vi "Lookup Channels.vi"(8 "error in (no error)":errorcluster, 11 "HTTP Command Bridge in":refnum<class "HTTP Command Bridge.lvclass">) -> (0 "error out":errorcluster, 3 "HTTP Command Bridge out":refnum<class "HTTP Command Bridge.lvclass">)   [LabVIEW 2020, in "Volatus.lvlib" / "HTTP Command Bridge.lvclass"]
uses:
  HTTP Command Bridge.lvclass
  HTTP Command Bridge.lvclass/HTTP Command Bridge.ctl
  Module/Module.lvclass
  VolatusAPI/VolatusAPI.lvclass
  Command Dest.ctl
  MessageQ/MessageQ.lvclass
  Command Info.ctl
  C:/dev/lv20CE/relink/lv-volatus/Volatus/Module/Module.lvclass
  C:/dev/lv20CE/relink/lv-volatus/Volatus/HTTP Command Bridge/HTTP Command Bridge.lvclass
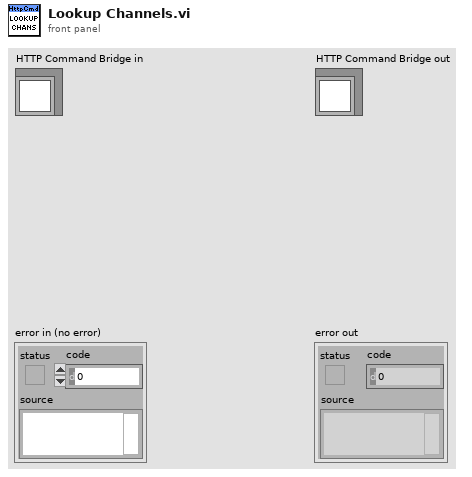
[diagram p1: front panel]
types:
  T1 = typedef "Volatus.lvlib/HTTP Command Bridge.lvclass/Command Info.ctl" = cluster{"Destination":T2, "Local Q":refnum<class "MessageQ.lvclass">, "Target":string, "Task":string}
  T2 = typedef "Volatus.lvlib/HTTP Command Bridge.lvclass/Command Dest.ctl" = enum16{"Local", "Remote"}
  T3 = typedef "VectoConfig.lvlib/Channel Info.ctl" = cluster{"Name":string, "Group":string, "Owning Node":string, "Owning Task":string, "Resource":string}
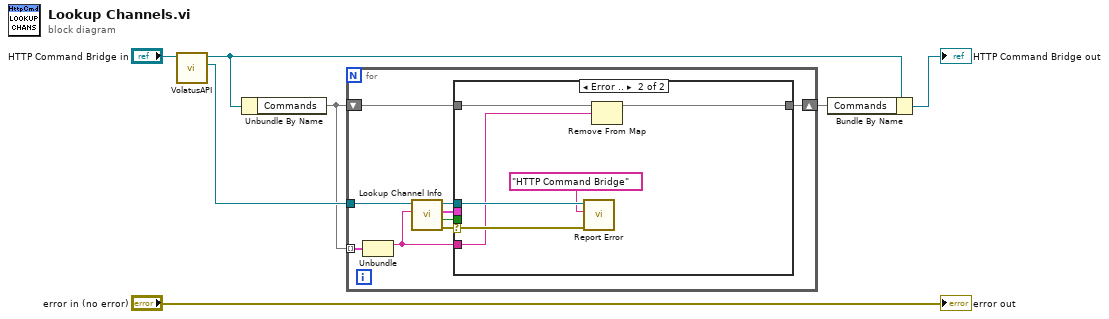
[diagram p0: block diagram]
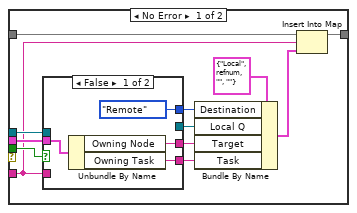
[diagram p2: hidden frame]
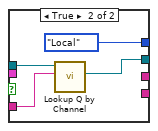
[diagram p3: hidden frame]
diagram:
  n1 = call "VolatusAPI.vi"("Module in"="HTTP Command Bridge in") -> ("VolatusAPI"=w6:refnum<class "VolatusAPI.lvclass">, "Module out"=w4:refnum<class "HTTP Command Bridge.lvclass">)  [unwired: 9 in]
  n2 = Unbundle By Name(w4) -> ("Commands"=w5:map{string, T1})
  n3 = for {
    tunnel: w6 -> [w16]
    shift-right: [w10] -> w3
    shift-left: w5 -> [w11]
    tunnel: w5 -> [w15] mode=indexing
    n4 = Unbundle(w15) -> ("Channel"=w9:string)  [unwired: 1 out]
    n5 = call "Lookup Channel Info.vi"("Channel Name"=w9, "VolatusAPI in"=w16) -> ("error out"=w8:errorcluster, "Local"=w13:bool, "Channel Info"=w12:T3, "VolatusAPI out"=w14:refnum<class "VolatusAPI.lvclass">)  [unwired: 5 in, 1 out]
    n6 = case shown="Error .." w8 {
      selector: w8 -> [_ w40]
      tunnel: w14 -> [w28 w42]
      tunnel: w13 -> [w27 _]
      tunnel: w12 -> [w26 _]
      tunnel: w11 -> [w25 w39]
      tunnel: [w21 w38] -> w10
      tunnel: w9 -> [w20 w37]
      frame No Error {
        n7 = case shown="False" w27 {
          tunnel: w28 -> [_ w36]
          tunnel: w20 -> [_ w35]
          tunnel: w26 -> [w31 _]
          tunnel: [Command_Dest."Remote" ("Command Dest") Command_Dest."Local" ("Command Dest")] -> w24
          tunnel: [_ w33] -> w19
          tunnel: [w30 _] -> w18
          tunnel: [w29 _] -> w17
          frame False {
            n8 = Unbundle By Name(w31) -> ("Owning Node"=w30:string, "Owning Task"=w29:string)
          }
          frame True {
            n9 = call "Lookup Q by Channel.vi"("Channel Name"=w35, "VolatusAPI in"=w36) -> ("MessageQ"=w33:refnum<class "MessageQ.lvclass">)  [unwired: 7 in, 2 out]
          }
        }
        n10 = Bundle By Name(cluster=T1 {"Destination"=enum."Local", "Local Q"=refnum, "Target"="", "Task"=""} ("value"), "Destination"=w24, "Local Q"=w19, "Target"=w18, "Task"=w17) -> (w22:T1)
        n11 = Insert Into Map(map in=w25, key=w20, value=w22) -> (map out=w21:map{string, T1})  [unwired: 2 out]
      }
      frame Error {
        n12 = call "Report Error.vi"("error in (no error)"=w40, "Context"="HTTP Command Bridge", "VolatusAPI in"=w42) -> ()  [unwired: 7 in, 2 out]
        n13 = Remove From Map(10:w37, 11:w39) -> (3:w38:map{string, T1})  [unwired: 2 out]
      }
    }
  }
  n14 = Bundle By Name(cluster=w4, "Commands"=w3) -> (→"HTTP Command Bridge out":refnum<class "HTTP Command Bridge.lvclass">)
  "error out" <- "error in (no error)"
